vi "pid_test.vi"() -> ()   [LabVIEW 2017]
uses:
  <vilib>/myRIO/Common/Instrument Driver Framework/myRIO v1.0/Encoder/typedefs/Encoder Signal Mode.ctl
  <vilib>/myRIO/Instrument Drivers/Onboard IO/Encoder/typedefs/Encoder Reference.ctl
  <vilib>/myRIO/Common/Instrument Driver Framework/Utilities/typedefs/myRIO Generic Hardware Reference.ctl
  <vilib>/myRIO/Common/Instrument Driver Framework/Utilities/typedefs/Hardware Version Enum.ctl
  <vilib>/myRIO/Common/Instrument Driver Framework/Utilities/typedefs/myRIO v1.0 Reference.ctl
  <vilib>/myRIO/Common/Instrument Driver Framework/Utilities/typedefs/Generic FPGA Reference.ctl
  <vilib>/myRIO/Common/Instrument Driver Framework/myRIO v1.0/Encoder/typedefs/Encoder Channels Enum.ctl
  <vilib>/myRIO/Common/Instrument Driver Framework/myRIO v1.0/Encoder/typedefs/Encoder Configuration v1.0.ctl
  <vilib>/userdefined/High Color/nirio_resource_hc.ctl
  <vilib>/myRIO/Common/Instrument Driver Framework/Utilities/vis/Is FPGA Ref Available.vi
  <vilib>/myRIO/Common/Instrument Driver Framework/myRIO v1.0/Encoder/vis/myRIO v1.1 Open Encoder.vi
  <vilib>/myRIO/Instrument Drivers/Onboard IO/Encoder/vis/Read.vi
  <vilib>/myRIO/Common/Instrument Driver Framework/Utilities/vis/Validate Channels.vi
  <vilib>/myRIO/Common/Instrument Driver Framework/myRIO v1.0/Encoder/vis/myRIO v1.0 Reserve Encoder.vi
  <vilib>/myRIO/Common/Instrument Driver Framework/myRIO v1.0/UART/vis/myRIO v1.0 Close UART.vi
  <vilib>/myRIO/Common/Instrument Driver Framework/myRIO v1.0/Encoder/vis/myRIO v1.0 Build MUX Configuration Encoder.vi
  <vilib>/myRIO/Common/Instrument Driver Framework/myRIO v1.0/Resource Manager/vis/myRIO v1.0 Reserve Channel List.vi
  <vilib>/myRIO/Common/Instrument Driver Framework/myRIO v1.0/Resource Manager/vis/myRIO v1.0 Create Configuration List.vi
  <vilib>/myRIO/Common/Instrument Driver Framework/myRIO v1.0/Resource Manager/vis/myRIO v1.0 Reserve Channel.vi
  <vilib>/myRIO/Common/Instrument Driver Framework/myRIO v1.0/Resource Manager/vis/myRIO v1.0 Unreserve Channel.vi
  <vilib>/myRIO/Common/Instrument Driver Framework/myRIO v1.0/Resource Manager/vis/myRIO v1.0 Build Mutex Name.vi
  <vilib>/Utility/VariantDataType/GetNumericInfo.vi
  <vilib>/Utility/error.llb/Error Cluster From Error Code.vi
  <vilib>/myRIO/Common/Instrument Driver Framework/myRIO v1.0/myRIO v1.1 Open.vi
  <vilib>/myRIO/Common/Instrument Driver Framework/Utilities/vis/IO Manager.vi
  <vilib>/myRIO/Common/Instrument Driver Framework/Utilities/vis/Configuration Manager.vi
  <vilib>/myRIO/Common/Instrument Driver Framework/myRIO v1.0/Resource Manager/vis/myRIO v1.0 Configure IO.vi
  <vilib>/myRIO/Common/Instrument Driver Framework/myRIO v1.0/myRIO v1.0 Close.vi
  <vilib>/myRIO/Common/Instrument Driver Framework/myRIO v1.0/Encoder/vis/myRIO v1.0 Configure Encoder.vi
  <vilib>/myRIO/Common/Instrument Driver Framework/myRIO v1.0/Encoder/vis/myRIO v1.0 Read Encoder.vi
  <vilib>/myRIO/Common/Instrument Driver Framework/Utilities/vis/FPGA Ref Manager.vi
  <vilib>/myRIO/Common/Instrument Driver Framework/myRIO v1.0/myRIO v1.0 Reset FPGA.vi
  <vilib>/myRIO/Common/Instrument Driver Framework/myRIO v1.0/IRQ/vis/myRIO v1.0 IRQ Info FGV.vi
  <vilib>/myRIO/Common/Instrument Driver Framework/myRIO v1.0/IRQ/vis/myRIO v1.0 Timer IRQ Info FGV.vi
  <vilib>/myRIO/Common/Instrument Driver Framework/myRIO v1.0/IRQ/vis/myRIO v1.0 ISR Agent.vi
  <vilib>/myRIO/Express VI/Onboard IO/Encoder/Encoder Express VI.xnode
  <vilib>/myRIO/Instrument Drivers/Onboard IO/Encoder/vis/myRIO Encoder Open.xnode
  <vilib>/myRIO/Common/Instrument Driver Framework/myRIO v1.0/Encoder/typedefs/Encoder Count Direction Enum.ctl
  <vilib>/myRIO/Instrument Drivers/Utilities/Utilities.lvlib
  <vilib>/myRIO/Instrument Drivers/Onboard IO/Encoder/Encoder.lvlib
panel:
  in  "stop":bool
  out "Waveform Chart":dbl(graph)
  in  "Speed":dbl(slide) scale=0.0..10.0
  out "thetadiff":dbl
  out "OUTPUT B":dbl(slide) scale=-10.0..10.0
  out "OUTPUT A":dbl(slide) scale=-10.0..10.0
  out "PID A":T1(graph)
  out "PID B":T1(graph)
  out "Setpoint A":dbl(slide) scale=-10.0..10.0
  out "Setpoint B":dbl(slide) scale=-10.0..10.0
  out "X, Y, BEARING":cluster{dbl, dbl, dbl}
  out "XY Graph":cluster{"X":dbl, "Y":dbl}[](graph)
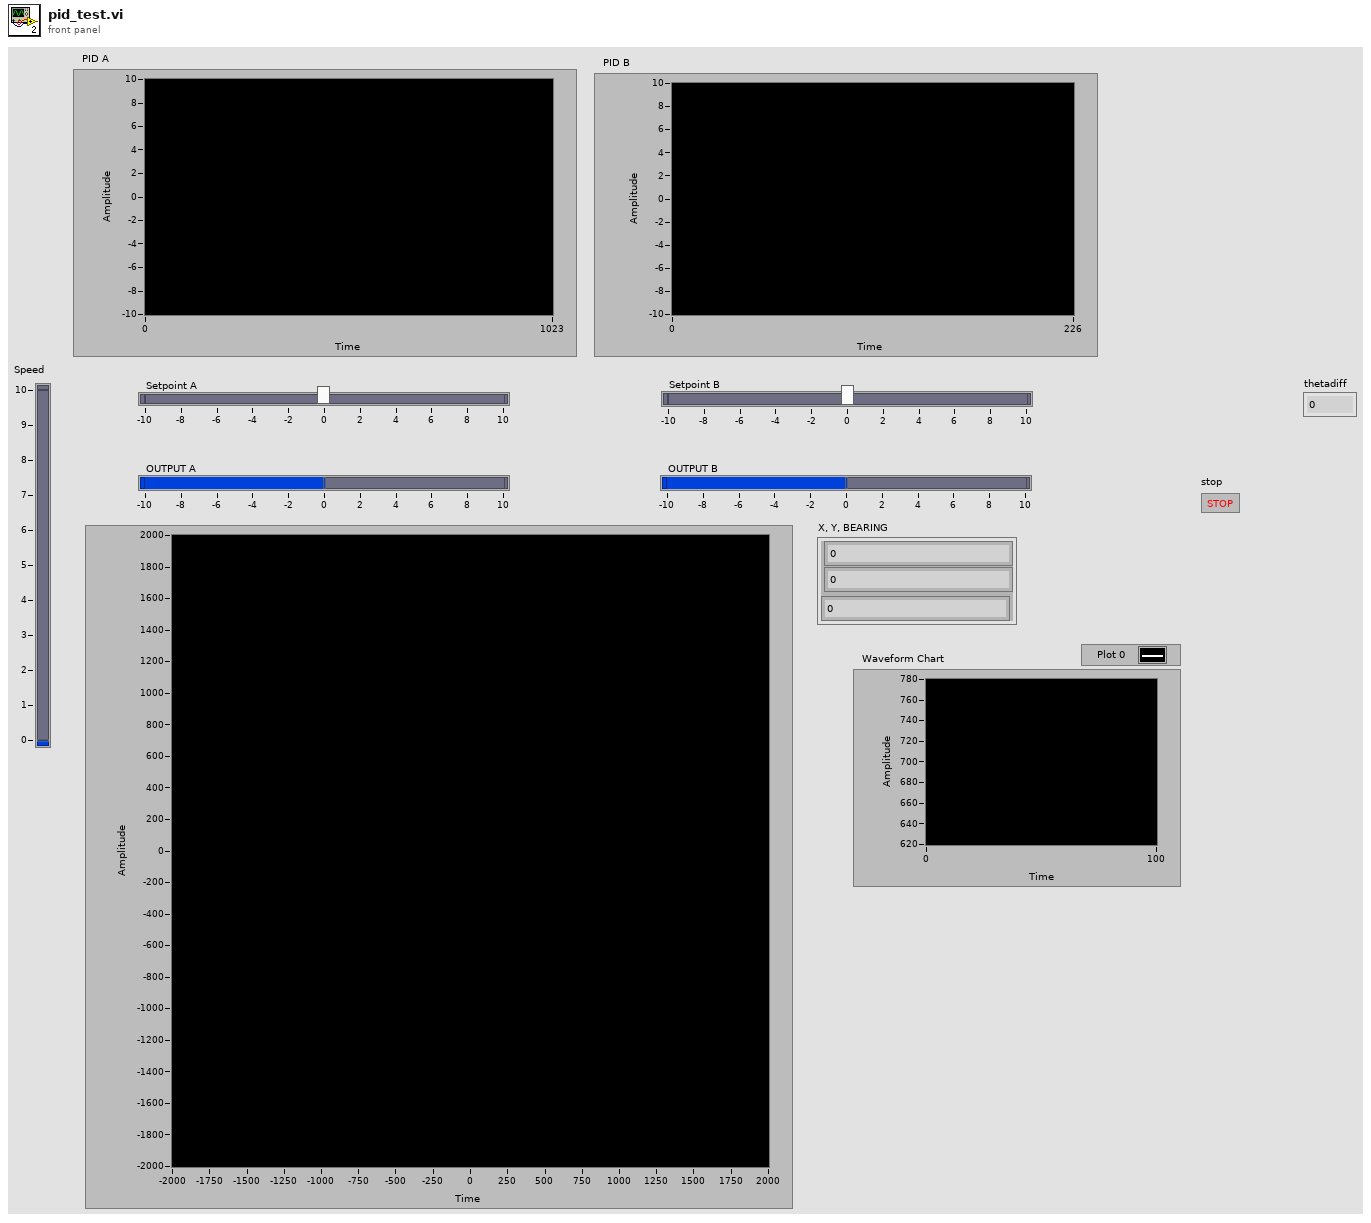
[diagram p1: front panel]
types:
  T1 = cluster{"Setpoint":dbl, "output":dbl, "dx/dt":dbl}
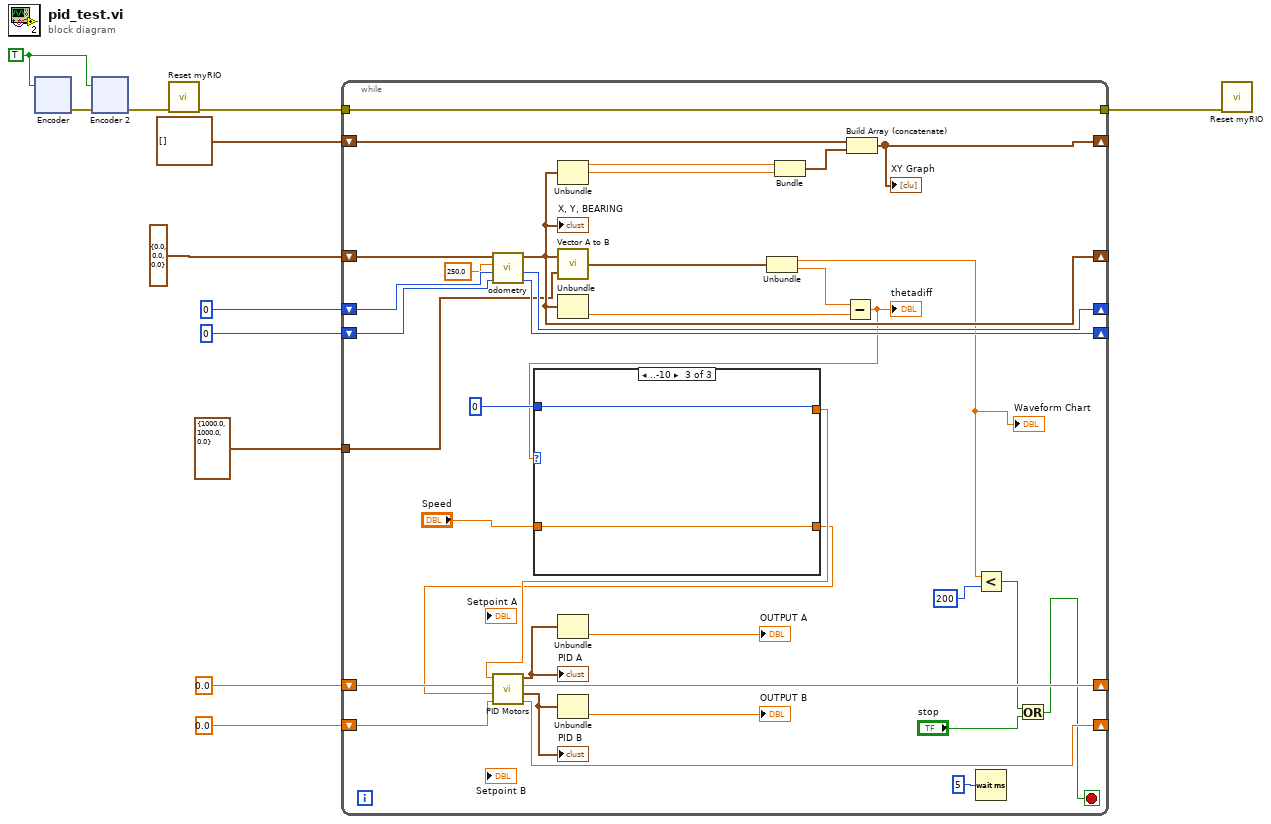
[diagram p0: block diagram]
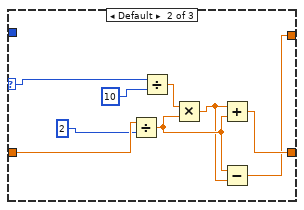
[diagram p3: hidden frame]
diagram:
  w5 = TRUE
  n1 = xnode "Encoder"("Reset Counter"=w5) -> ("error out"=w6:errorcluster)  [unwired: 1 in, 3 out]
  n2 = xnode "Encoder 2"("error in (no error)"=w6, "Reset Counter"=w5) -> ("error out"=w7:errorcluster)  [unwired: 3 out]
  n3 = call <vilib>:"Reset myRIO.vi"("error in (no error)"=w7) -> ("error out"=w11:errorcluster)  [unwired: 10 in]
  n4 = while {
    shift-right: [w27] -> _
    shift-left: cluster{dbl, dbl, dbl} {0.0, 0.0, 0.0} ("X, Y, BEARING") -> [w48]
    shift-right: [w46] -> _
    shift-left: 0 ("ENCA OUT") -> [w47]
    shift-right: [w45] -> _
    shift-left: 0 ("ENCB OUT") -> [w44]
    shift-right: [w39] -> _
    shift-left: cluster{dbl, dbl}[] [] -> [w40]
    tunnel: w11 -> [w32]
    shift-right: [w34] -> _
    shift-left: 0.0 ("output A") -> [w35]
    shift-right: [w37] -> _
    shift-left: 0.0 ("output B") -> [w36]
    tunnel: [w32] -> w2
    tunnel: cluster{dbl, dbl, dbl} {1000.0, 1000.0, 0.0} ("X, Y, BEARING") -> [w13]
    stop <- w14 stop-if-true
    n5 = call "odometry.vi"("ENCB in"=w44, "ENCA in"=w47, "wheelbase"=250.0, "Position"=w48) -> ("ENCB OUT"=w45:i32, "ENCA OUT"=w46:i32, "X, Y, BEARING"=w27:cluster{dbl, dbl, dbl})  [unwired: 4 in]
    "X, Y, BEARING" <- w27
    n6 = Unbundle(w27) -> (w43:dbl, w42:dbl)  [unwired: 1 out]
    n7 = call "Vector A to B.vi"("Destination"=w13, "Current"=w27) -> ("vector"=w26:cluster{dbl, "Bearing":dbl})
    n8 = Unbundle(w27) -> (w24:dbl)  [unwired: 2 out]
    n9 = Unbundle(w26) -> (w17:dbl, "Bearing"=w25:dbl)
    "Waveform Chart" <- w17
    n10 = Bundle(w43, w42) -> (w41:cluster{dbl, dbl})  [unwired: 1 in]
    n11 = Subtract(x=w25, y=w24) -> (x-y=w19:dbl)
    "thetadiff" <- w19
    n12 = case shown="..-10" w19 {
      selector: w19 -> [_ w56 _]
      tunnel: "Speed" -> [w50 w59 w61]
      tunnel: [w49 w52 w61] -> w20
      tunnel: [w50 w51 w60] -> w21
      tunnel: 0 -> [w49 _ w60]
      frame 10.. {
      }
      frame Default {
        n13 = Divide(x=w59, y=2) -> (x/y=w54:dbl)
        n14 = Divide(x=w56, y=10) -> (x/y=w55:dbl)
        n15 = Multiply(x=w55, y=w54) -> (x*y=w53:dbl)
        n16 = Add(x=w53, y=w54) -> (x+y=w52:dbl)
        n17 = Subtract(x=w54, y=w53) -> (x-y=w51:dbl)
      }
      frame ..-10 {
      }
    }
    n18 = call "PID Motors.vi"("input B"=w36, "Speed B"=w20, "input A"=w35, "Speed A"=w21) -> ("output B"=w37:dbl, "Speed B0"=w30:T1, "output A"=w34:dbl, "Speed A0"=w31:T1)
    "PID B" <- w30
    "PID A" <- w31
    n19 = Unbundle(w31) -> ("dx/dt"=→"OUTPUT A":dbl)  [unwired: 2 out]
    n20 = Unbundle(w30) -> ("dx/dt"=→"OUTPUT B":dbl)  [unwired: 2 out]
    n21 = Build Array (concatenate)(w40, w41) -> (w39:cluster{dbl, dbl}[])
    "XY Graph" <- w39
    n22 = Less?(x=w17, y=200) -> (x < y?=w16:bool)
    n23 = Wait (ms)(milliseconds to wait=5 ("ENCB OUT")) -> ()  [unwired: 1 out]
    n24 = Or(x=w16, y="stop") -> (x .or. y?=w14:bool)
  }
  n25 = call <vilib>:"Reset myRIO.vi"("error in (no error)"=w2) -> ()  [unwired: 10 in, 1 out]
